vi "HISW-TimeScope.vi"(2 "Time":timestamp) -> (7 "Valid?":bool)   [LabVIEW 2020, in "Sgraph_lib_V1.lvlib" / "HISW.lvclass"]
doc: "Check if a sample is within the allowed time limit.\nIf outside this limit: the time value is considered to be an error."
uses:
  HISW.lvclass
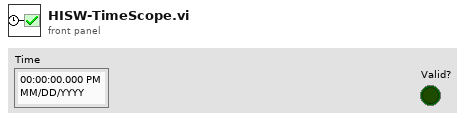
[diagram p1: front panel]
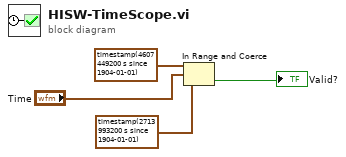
[diagram p0: block diagram]
diagram:
  n1 = In Range and Coerce(upper limit=timestamp(4607449200 s since 1904-01-01) ("y"), x="Time", lower limit=timestamp(2713993200 s since 1904-01-01) ("y")) -> (In Range?=→"Valid?":bool)  [unwired: 1 out]
